vi "destroy.vi"(8 "error in (no error)":errorcluster, 11 "TaskMock in":refnum<class "TaskMock.lvclass">) -> (0 "error out":errorcluster)   [LabVIEW 2023, in "TaskMock.lvclass"]
uses:
  TaskMock.lvclass
  TaskMock.lvclass/TaskMock.ctl
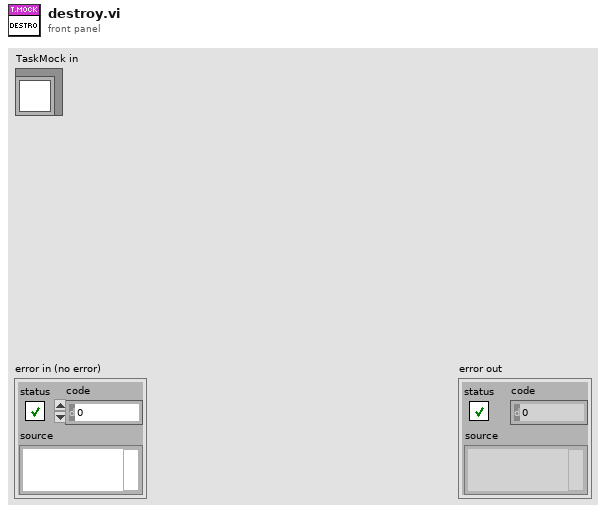
[diagram p1: front panel]
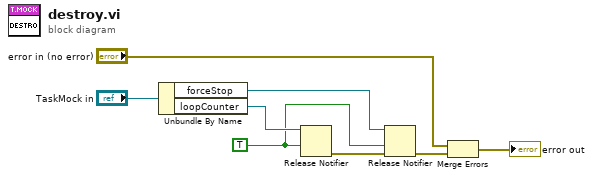
[diagram p0: block diagram]
diagram:
  w1 = TRUE ("force destroy? (F)")
  n1 = Unbundle By Name("TaskMock in") -> ("forceStop"=w2:refnum<notifier>, "loopCounter"=w7:refnum<notifier>)
  n2 = Release Notifier(notifier=w7, force destroy? (F)=w1) -> (error out=w4:errorcluster)  [unwired: 1 in, 2 out]
  n3 = Release Notifier(notifier=w2, force destroy? (F)=w1, error in (no error)=w4) -> (error out=w3:errorcluster)  [unwired: 2 out]
  n4 = Merge Errors("error in (no error)", w3) -> (→"error out":errorcluster)
